vi "Get Queueu FPGA.vi"(8 "error in (no error)":errorcluster) -> (0 "error out":errorcluster, 3 "Error Queue":refnum<queue>)   [LabVIEW 2023, in "FPGA.lvlib"]
uses:
  FPGA.lvlib
  Downloads/ATM (100528-01)/ATM (100528-01)/Omi-One Solution/Inner Process Communication/States Queues FGV.ctl
  Downloads/ATM (100528-01)/ATM (100528-01)/Omi-One Solution/Inner Process Communication/Innes Process Communication.lvlib
  Internal Communication/Internal Communication.lvlib
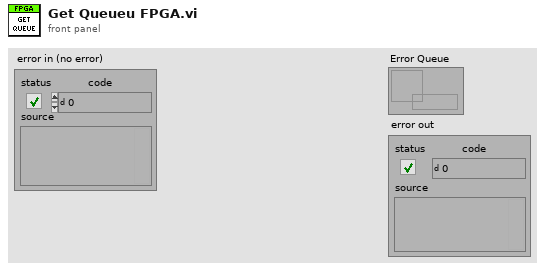
[diagram p1: front panel]
types:
  T1 = typedef "Innes Process Communication.lvlib/States Queues FGV.ctl" = enum16{"Create Queues", "Get Queues", "Destroy Queues"}
  T2 = typedef "Internal Communication.lvlib/Queues Control.ctl" = cluster{"Heart":refnum<queue>, "FPGA":refnum<queue>, "Encoder":refnum<queue>, "Decoder":refnum<queue>, "Error":refnum<queue>, "UI":refnum<queue>}
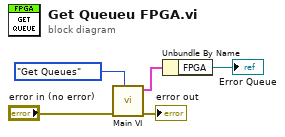
[diagram p0: block diagram]
diagram:
  n1 = call "Main VI.vi"("Enum"=States_Queues_FGV."Get Queues", "error in (no error)"="error in (no error)") -> ("error out"=→"error out":errorcluster, "Queues"=w4:T2)  [unwired: 8 in]
  n2 = Unbundle By Name(w4) -> ("FPGA"=→"Error Queue":refnum<queue>)
